vi "AllOff.vi"(8 "RightIn":dbl, 9 "LeftIn":dbl, 10 "WandIn":dbl, 11 "ButtonIn":bool) -> (0 "RightOut":dbl, 1 "LeftOut":dbl, 2 "WandOut":dbl, 3 "Compressor":bool)   [LabVIEW 2015]
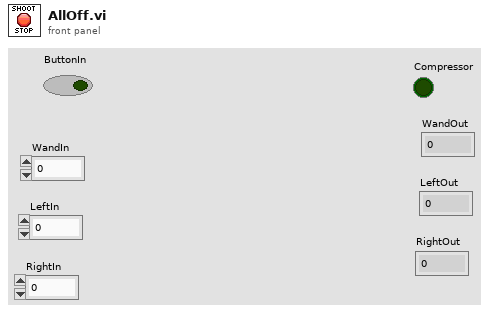
[diagram p1: front panel]
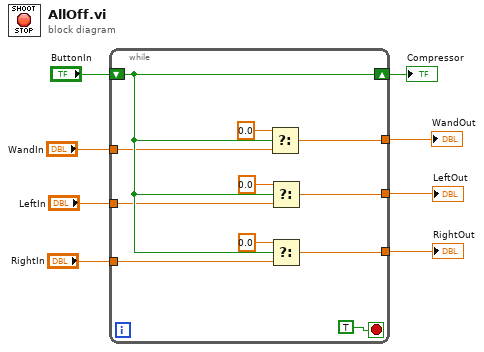
[diagram p0: block diagram]
diagram:
  n1 = while {
    shift-right: [w17] -> w7
    shift-left: "ButtonIn" -> [w17]
    tunnel: [w18] -> w6
    tunnel: [w16] -> w5
    tunnel: [w15] -> w4
    tunnel: "RightIn" -> [w11]
    tunnel: "LeftIn" -> [w10]
    tunnel: "WandIn" -> [w9]
    stop <- TRUE stop-if-true
    n2 = Select(t=0.0, s=w17, f=w9) -> (s? t:f=w15:dbl)
    n3 = Select(t=0.0, s=w17, f=w10) -> (s? t:f=w18:dbl)
    n4 = Select(t=0.0, s=w17, f=w11) -> (s? t:f=w16:dbl)
  }
  "Compressor" <- w7
  "WandOut" <- w4
  "LeftOut" <- w6
  "RightOut" <- w5
